vi "PostEventsToDatabase.vi"(8 "error in (no error)":errorcluster) -> (0 "error out":errorcluster)   [LabVIEW 2014, in "FIRST Events API.lvlib"]
uses:
  FIRST Events API.lvlib
  Backend/source/VI Source/FRCts20_Backend_API/FRCts20_Backend_API_EventRoot.ctl
  Backend/source/VI Source/FRCts20_Backend_API/FRCts20_Backend_API_Command_EventRoot.ctl
  Backend/source/VI Source/FRCts20_Backend_API/FRCts20_Backend_API_EventRoot.vi
  Backend/source/VI Source/FRCts20_Backend_API/FRCts20_Backend_API.lvlib
panel:
  out "Items added to database":i32
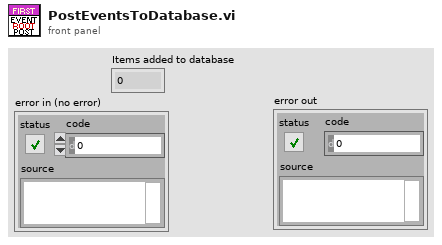
[diagram p1: front panel]
types:
  T1 = typedef "FRCts20_Backend_API.lvlib/FRCts20_Backend_API_EventRoot.ctl" = cluster{"Event":cluster{"Event Index":u32, "EventID":u32, "EventSubtype":string, "EventSubtypeID":u32, "DistrictCode":string, "DistrictID":u32, "Event Name":string, "Venue":string, "City":string, "StateProvince":string, "Country":string, "Start Time":timestamp, "End Time":timestamp, "Year":u32, "NumberOfTeams":u32, "URLTeamlist":string, "EventCode":string, "OpenIssues":u8, "IsLive":bool}[], "APIReturn":string}
  T2 = cluster{"Event Index":u32, "EventID":u32, "EventSubtype":string, "EventSubtypeID":u32, "DistrictCode":string, "DistrictID":u32, "Event Name":string, "Venue":string, "City":string, "StateProvince":string, "Country":string, "Start Time":timestamp, "End Time":timestamp, "Year":u32, "NumberOfTeams":u32, "URLTeamlist":string, "EventCode":string, "OpenIssues":u8, "IsLive":bool}[]
  T3 = typedef "FRCts20_Backend_API.lvlib/FRCts20_Backend_API_Command_EventRoot.ctl" = string
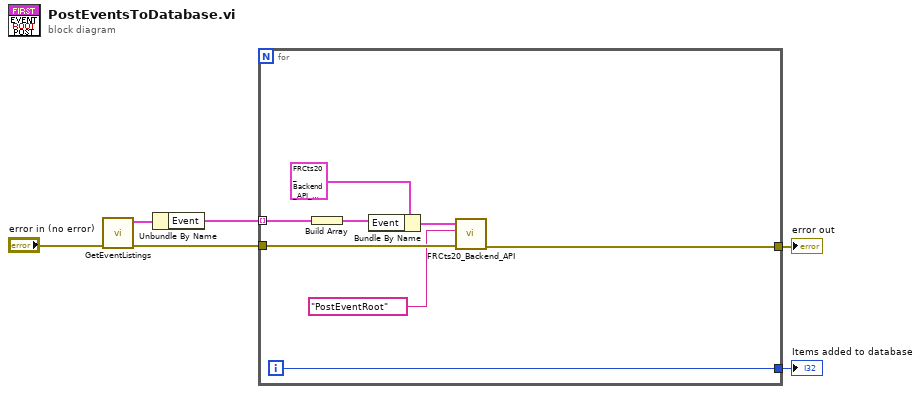
[diagram p0: block diagram]
diagram:
  n1 = call "GetEventListings.vi"("error in (no error)"="error in (no error)") -> ("error out"=w4:errorcluster, "output cluster"=w6:T1)  [unwired: 8 in, 1 out]
  n2 = Unbundle By Name(w6) -> ("Event"=w5:T2)
  n3 = for {
    tunnel: w5 -> [w13] mode=indexing
    tunnel: w4 -> [w10]
    tunnel: [w9] -> w3
    tunnel: [w8] -> w2
    i -> [w8]
    n4 = Build Array(w13) -> (w12:T2)
    n5 = Bundle By Name(cluster=T1 data[22150B] ("output cluster"), "Event"=w12) -> (w11:T1)
    n6 = call-poly "FRCts20_Backend_API.vi"("error in (no error)"=w10, "Message"=T3 "PostEventRoot", "EventRoot In"=w11) -> ("error out"=w9:errorcluster)  [unwired: 6 in, 2 out]
  }
  "error out" <- w3
  "Items added to database" <- w2
